vi "Append String to Array.vi"(9 "array":string[](array[string]), 10 "name":string) -> (2 "result":string[](array[string]))   [LabVIEW 2011, in "GripsMaster.lvclass"]
uses:
  GripsMaster.lvclass
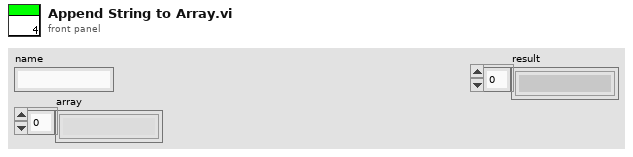
[diagram p1: front panel]
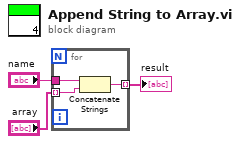
[diagram p0: block diagram]
diagram:
  n1 = for {
    tunnel: "name" -> [w6]
    tunnel: [w5] -> w1 mode=indexing
    tunnel: "array" -> [w4] mode=indexing
    n2 = Concatenate Strings(w6, w4) -> (w5:string)
  }
  "result" <- w1
